vi "check_queue.vi"(7 "State":T1=enum."End", 8 "Error In":errorcluster, 10 "DaQ QMH":refnum<queue>, 11 "Calibrator Queue":refnum<queue>) -> (0 "Error Out":errorcluster)   [LabVIEW 2021, in "Main.lvlib" / "Main_Programs_SubVIs.lvlib"]
doc: "This subVi is used to control the QMH and the notifier."
uses:
  Main_Programs_SubVIs.lvlib
  Tipski Definicii/QMH_Daq_States.ctl
  Tipski Definicii/Kalibrator_Sostojbi.ctl
  Polymorphic/Enq_Calibrator_QMH.vi
  Polymorphic/Prev_Calibrator_QMH.vi
  Polymorphic/Enq_DaQ_QMH.vi
  Polymorphic/Queues.lvlib
panel:
  # "Output"
  # "Input"
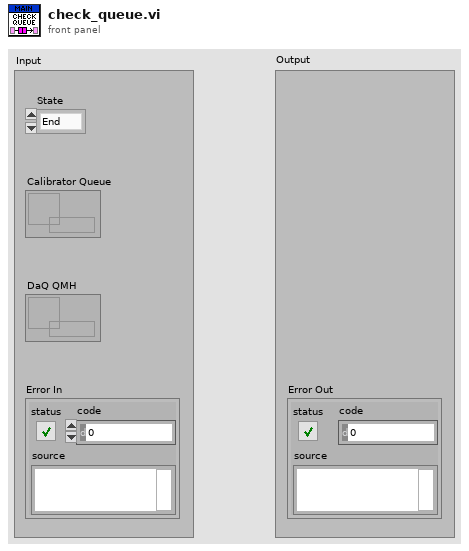
[diagram p1: front panel]
types:
  T1 = typedef "Kalibrator_Sostojbi.ctl" = enum16{"Init", "Idle", "Standby", "Operate ", "End"}
  T2 = typedef "QMH_Daq_States.ctl" = enum16{"Idle", "Start DaQ", "DaQ", "Generate Message", "Stop DaQ", "End"}
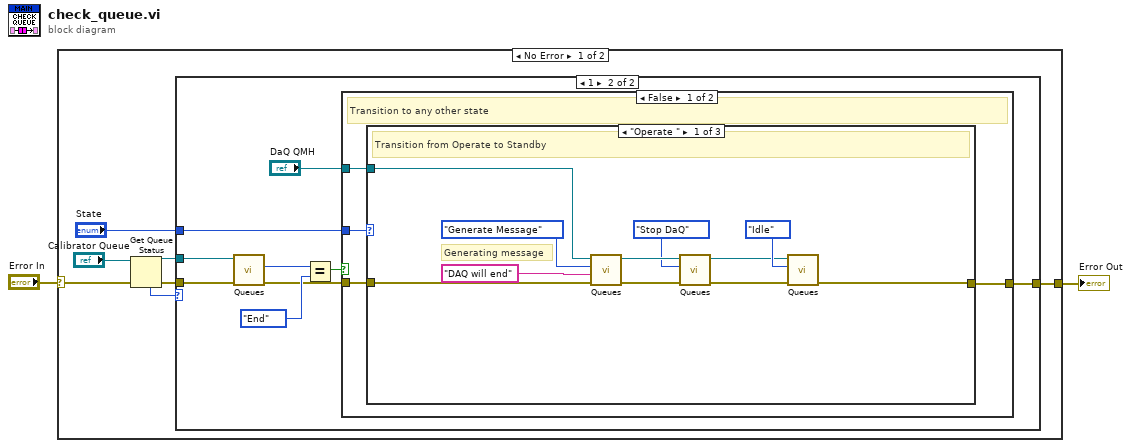
[diagram p0: block diagram]
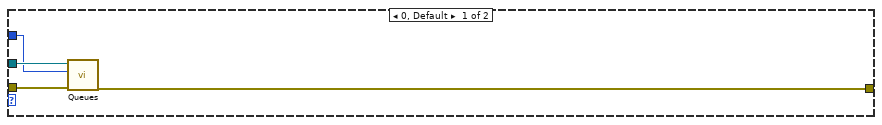
[diagram p2: hidden frame]
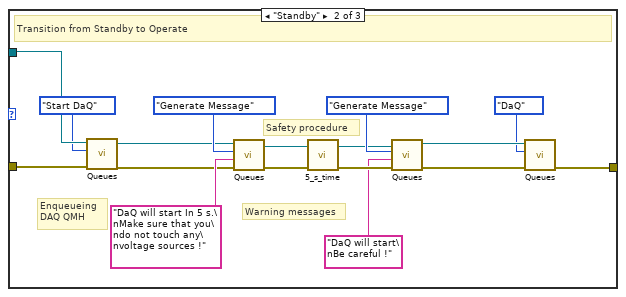
[diagram p3: hidden frame]
diagram:
  n1 = case shown="No Error" "Error In" {
    selector: "Error In" -> [w5 w56]
    tunnel: [w9 w56] -> w2
    frame No Error {
      n2 = Get Queue Status(queue="Calibrator Queue", error in (no error)=w5) -> (queue out=w7:refnum<queue>, error out=w8:errorcluster, # elements in queue=w6:i32)  [unwired: 1 in, 5 out]
      n3 = case shown="1" w6 {
        tunnel: w7 -> [w11 w18]
        tunnel: w8 -> [w13 w19]
        tunnel: [w12 w22] -> w9
        tunnel: "State" -> [w10 w21]
        frame 0, Default {
          n4 = call-poly "Queues.vi"("Error In"=w13, "Instruction"=w10, "Queue In"=w11) -> ("Error Out"=w12:errorcluster)  [unwired: 7 in, 1 out]
        }
        frame 1 {
          n5 = call-poly "Queues.vi"("Error In"=w19, "Queue In"=w18) -> ("Error Out"=w14:errorcluster, "Instruction"=w17:T1)  [unwired: 6 in, 2 out]
          n6 = Equal?(x=w17, y=Kalibrator_Sostojbi."End") -> (x = y?=w16:bool)
          n7 = case shown="False" w16 {
            tunnel: w14 -> [w26 w55]
            tunnel: [w25 w55] -> w22
            tunnel: w21 -> [w24 _]
            tunnel: "DaQ QMH" -> [w23 _]
            frame False {
              # "Transition to any other state"
              n8 = case shown="\"Operate \"" w24 {
                tunnel: w26 -> [w34 w53 w54]
                tunnel: [w29 w40 w54] -> w25
                tunnel: w23 -> [w37 w52 _]
                frame "Operate " {
                  # "Generating message"
                  # "Transition from Operate to Standby"
                  n9 = call-poly "Queues.vi"("Error In"=w34, "Message"="DAQ will end", "Instruction"=QMH_Daq_States."Generate Message", "Queue In"=w37) -> ("Error Out"=w33:errorcluster, "Queue Out"=w32:refnum<queue>)  [unwired: 6 in]
                  n10 = call-poly "Queues.vi"("Error In"=w33, "Instruction"=QMH_Daq_States."Stop DaQ", "Queue In"=w32) -> ("Error Out"=w27:errorcluster, "Queue Out"=w28:refnum<queue>)  [unwired: 7 in]
                  n11 = call-poly "Queues.vi"("Error In"=w27, "Instruction"=QMH_Daq_States."Idle", "Queue In"=w28) -> ("Error Out"=w29:errorcluster)  [unwired: 7 in, 1 out]
                }
                frame "Standby" {
                  # "Safety procedure"
                  # "Enqueueing \nDAQ QMH"
                  # "Warning messages"
                  # "Transition from Standby to Operate"
                  n12 = call-poly "Queues.vi"("Error In"=w53, "Instruction"=QMH_Daq_States."Start DaQ", "Queue In"=w52) -> ("Error Out"=w43:errorcluster, "Queue Out"=w42:refnum<queue>)  [unwired: 7 in]
                  n13 = call-poly "Queues.vi"("Error In"=w43, "Message"="DaQ will start In 5 s.\nMake sure that you\ndo not touch any\nvoltage sources !", "Instruction"=QMH_Daq_States."Generate Message", "Queue In"=w42) -> ("Error Out"=w48:errorcluster, "Queue Out"=w47:refnum<queue>)  [unwired: 6 in]
                  n14 = call "5_s_time.vi"("Error In"=w48) -> ("Error Out"=w50:errorcluster)  [unwired: 10 in]
                  n15 = call-poly "Queues.vi"("Error In"=w50, "Message"="DaQ will start\nBe careful !", "Instruction"=QMH_Daq_States."Generate Message", "Queue In"=w47) -> ("Error Out"=w41:errorcluster, "Queue Out"=w39:refnum<queue>)  [unwired: 6 in]
                  n16 = call-poly "Queues.vi"("Error In"=w41, "Instruction"=QMH_Daq_States."DaQ", "Queue In"=w39) -> ("Error Out"=w40:errorcluster)  [unwired: 7 in, 1 out]
                }
                frame "Idle", Default {
                  # "Default case for no bugging"
                }
              }
            }
            frame True {
              # "Transiton to end"
            }
          }
        }
      }
    }
    frame Error {
    }
  }
  "Error Out" <- w2
